vi "2Ddistance.vi"(8 "error in (no error)":errorcluster, 10 "Location2":cluster{"X":dbl, "Y":dbl}, 11 "Location1":cluster{"X":dbl, "Y":dbl}) -> (0 "error out":errorcluster, 3 "Distance":dbl)   [LabVIEW 2009, in "OccupancyMap.lvclass"]
uses:
  OccupancyMap.lvclass
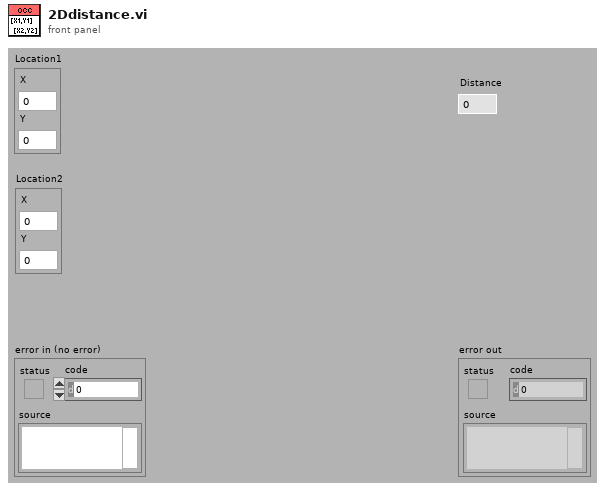
[diagram p1: front panel]
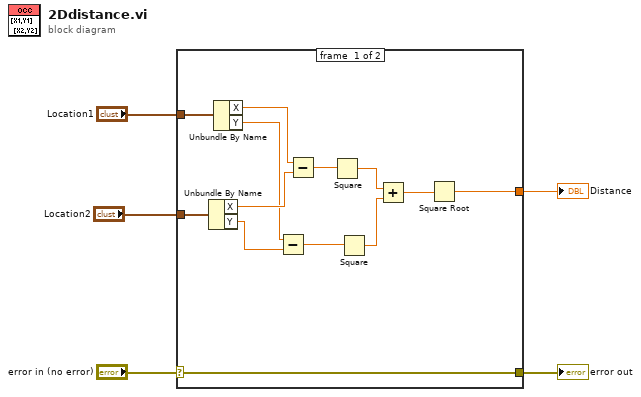
[diagram p0: block diagram]
diagram:
  n1 = case shown="Error" "error in (no error)" {
    selector: "error in (no error)" -> [w18 w19]
    tunnel: [w18 w19] -> w4
    tunnel: "Location1" -> [w17 _]
    tunnel: "Location2" -> [w16 _]
    tunnel: [w6 _] -> w1
    frame #0 {
      n2 = Unbundle By Name(w16) -> ("X"=w14:dbl, "Y"=w12:dbl)
      n3 = Unbundle By Name(w17) -> ("X"=w15:dbl, "Y"=w13:dbl)
      n4 = Subtract(x=w13, y=w12) -> (x-y=w10:dbl)
      n5 = Subtract(x=w15, y=w14) -> (x-y=w11:dbl)
      n6 = Square(x=w11) -> (x^2=w9:dbl)
      n7 = Square(x=w10) -> (x^2=w8:dbl)
      n8 = Add(x=w9, y=w8) -> (x+y=w7:dbl)
      n9 = Square Root(x=w7) -> (sqrt(x)=w6:dbl)
    }
    frame #1 {
    }
  }
  "error out" <- w4
  "Distance" <- w1
